vi "Write Last Waveform.vi"(8 "error in (no error)":errorcluster, 9 "Last Waveform":waveform(dbl), 10 "Channel":i32, 11 "Scope Base in":refnum<class "Scope Base.lvclass">) -> (0 "error out":errorcluster, 3 "Scope Base out":refnum<class "Scope Base.lvclass">)   [LabVIEW 2023, in "Scope Base.lvlib" / "Scope Base.lvclass"]
uses:
  Scope Base.lvclass
  Scope Base.lvclass/Scope Base.ctl
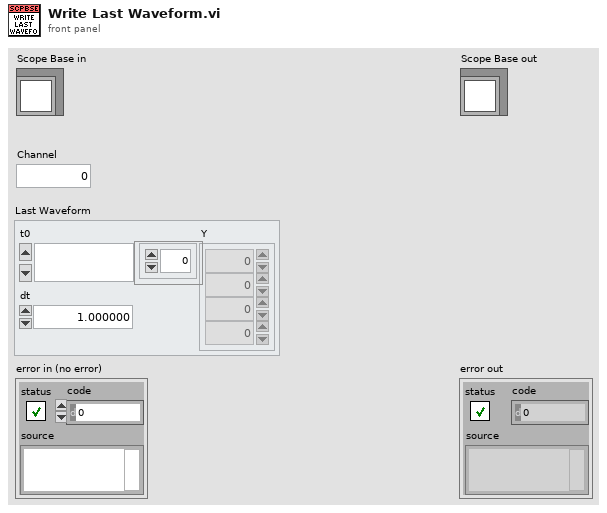
[diagram p1: front panel]
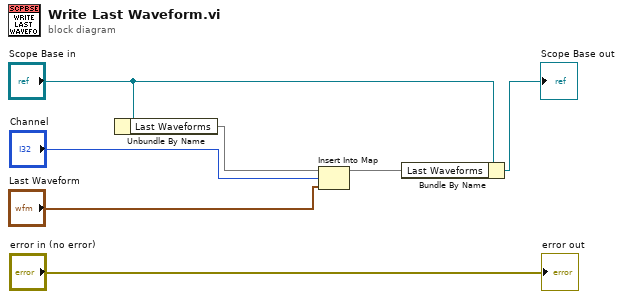
[diagram p0: block diagram]
diagram:
  n1 = Unbundle By Name("Scope Base in") -> ("Last Waveforms"=w4:map{i32, waveform(dbl)})
  n2 = Insert Into Map(map in=w4, key="Channel", value="Last Waveform") -> (map out=w3:map{i32, waveform(dbl)})  [unwired: 2 out]
  n3 = Bundle By Name(cluster="Scope Base in", "Last Waveforms"=w3) -> (→"Scope Base out":refnum<class "Scope Base.lvclass">)
  "error out" <- "error in (no error)"
